vi "ImageCode.vi"() -> ()   [LabVIEW 2012]
uses:
  <vilib>/Rock Robotics/WPI/Camera/WPI_CameraImageSize.ctl
panel:
  out "Image Error Message":string="Timeout in Camera Communications"
  in  "Viewer":enum32{"Camera Image"}(tab)
  in  "Video Enable":bool=TRUE
  out "Output String":string="!195,#END"
  out "Length":i32=9
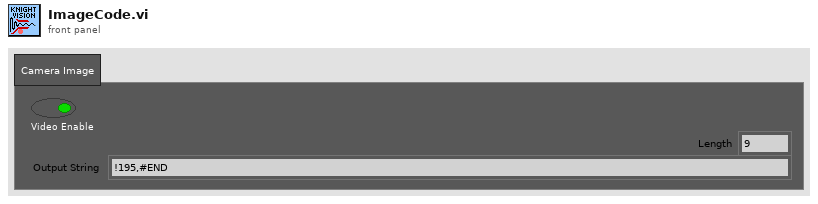
[diagram p1: front panel]
types:
  T1 = typedef "Image Type" = u32
  T2 = typedef "IMAQ Image.ctl" = refnum<image>
  T3 = cluster{"Left":i32, "Top":i32, "Right":i32, "Bottom":i32}
  T4 = typedef "WPI_CameraImageSize.ctl" = enum16{"640x480", "320x240", "160x120"}
  T5 = cluster{"fps":i32, "compression":i32, "Image Size":T4}
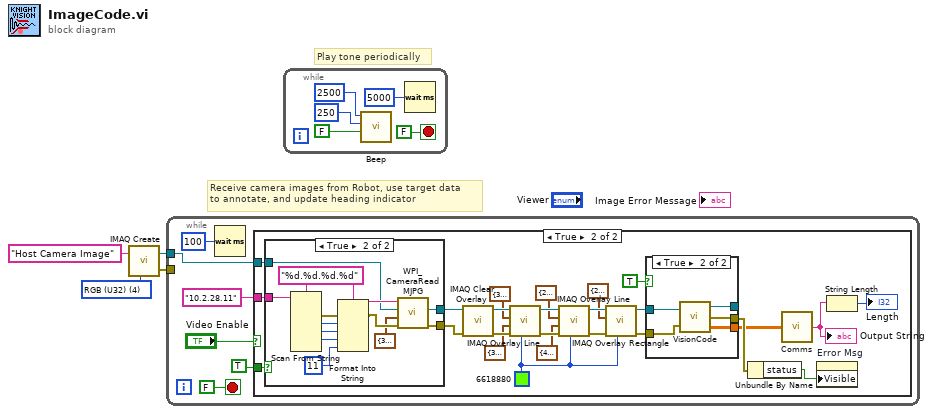
[diagram p0: block diagram]
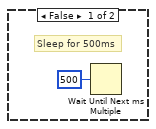
[diagram p2: hidden frame]
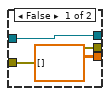
[diagram p3: hidden frame]
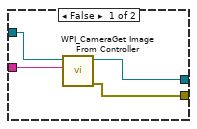
[diagram p4: hidden frame]
diagram:
  w4 = T1 4 items=["Grayscale (U8)", "Grayscale (I16)", "Grayscale (SGL)", "Complex (CSG)", "RGB (U32)", "HSL (U32)", "RGB (U64)"] ("Image Type")
  # "Play tone periodically"
  # "Receive camera images from Robot, use target data\nto annotate, and update heading indicator"
  n1 = call "IMAQ Create"("Image Name"="Host Camera Image", "Image Type"=w4) -> ("New Image"=w2:T2, "error out"=w1:errorcluster)  [unwired: 2 in, 1 out]
  n2 = while {
    tunnel: w2 -> [w8]
    tunnel: w1 -> [_]
    stop <- FALSE stop-if-true
    n3 = Wait (ms)(milliseconds to wait=u32 100) -> ()  [unwired: 1 out]
    n4 = case shown="True" "Video Enable" {
      tunnel: "10.2.28.11" ("Robot IP Address") -> [_ w36]
      tunnel: w8 -> [_ w35]
      tunnel: TRUE -> [_ w32]
      frame False {
        # "Sleep for 500ms"
        n5 = Wait Until Next ms Multiple(millisecond multiple=u32 500) -> ()  [unwired: 1 out]
      }
      frame True {
        w16 = u32 6618880 ("Color")
        n6 = case shown="True" w32 {
          tunnel: w35 -> [w47 w55]
          tunnel: [w45 w53] -> w12
          tunnel: [w46 w54] -> w33
          tunnel: w36 -> [w48 w58]
          frame False {
            n7 = call <vilib>:"WPI_CameraGet Image From Controller.vi"("Controller Address"=w48, "Image"=w47) -> ("error out"=w45:errorcluster, "Image Out"=w46:T2)  [unwired: 2 in, 6 out]
          }
          frame True {
            w50 = "%d.%d.%d.%d" ("format string")
            n8 = Scan From String(format string=w50, input string=w58) -> (error out=w57:errorcluster, output 1=w59:i32, output 2=w60:i32, output 3=w61:i32)  [unwired: 2 in, 7 out]
            n9 = Format Into String(format string=w50, error in=w57, w59, w60, w61, 11 ("IP Suffix:")) -> (resulting string=w56:string, error out=w52:errorcluster)  [unwired: 1 in]
            n10 = call <vilib>:"WPI_CameraRead MJPG.vi"("error in"=w52, "Camera Settings"=T5 {"fps"=30, "compression"=30, "Image Size"=enum."640x480"}, "Image"=w55, "address"=w56) -> ("error out"=w53:errorcluster, "Image Out"=w54:T2)  [unwired: 5 in, 1 out]
          }
        }
        n11 = call "IMAQ Clear Overlay"("error in (no error)"=w12, "Image"=w33) -> ("error out"=w30:errorcluster, "Image Out"=w31:T2)  [unwired: 1 in, 7 out]
        n12 = call "IMAQ Overlay Line"("Color"=w16, "error in (no error)"=w30, "End Point"=cluster{"X":i32, "Y":i32} {"X"=320, "Y"=480}, "Start Point"=cluster{"X":i32, "Y":i32} {"X"=320, "Y"=0}, "Image"=w31) -> ("error out"=w26:errorcluster, "Image Out"=w27:T2)  [unwired: 5 in]
        n13 = call "IMAQ Overlay Line"("Color"=w16, "error in (no error)"=w26, "End Point"=cluster{"X":i32, "Y":i32} {"X"=420, "Y"=240}, "Start Point"=cluster{"X":i32, "Y":i32} {"X"=220, "Y"=240}, "Image"=w27) -> ("error out"=w22:errorcluster, "Image Out"=w23:T2)  [unwired: 5 in]
        n14 = call "IMAQ Overlay Rectangle"("Color"=w16, "error in (no error)"=w22, "Rectangle"=T3 {"Left"=270, "Top"=190, "Right"=370, "Bottom"=290}, "Image"=w23) -> ("error out"=w20:errorcluster, "Image Out"=w18:T2)  [unwired: 6 in]
        n15 = case shown="True" TRUE {
          tunnel: w20 -> [w38 w44]
          tunnel: [w38 w41] -> w19
          tunnel: w18 -> [w39 w43]
          tunnel: [w39 w42] -> _
          tunnel: [dbl[][] [] ("Particle Measurements (Pixels)") w40] -> w15
          frame False {
          }
          frame True {
            n16 = call "VisionCode.vi"("Image Src"=w43, "error in (no error)"=w44) -> ("Image Out"=w42:T2, "error out"=w41:errorcluster, "Particle Measurements (Pixels)"=w40:dbl[][])
          }
        }
        n17 = Unbundle By Name(w19) -> ("status"=w34:bool)
        n18 = call "Comms.vi"("Array"=w15) -> ("String"=w14:string)
        "Output String" <- w14
        n19 = property on="Error Msg" class="Str"("Visible"=w34) -> ()  [unwired: 2 in, 2 out]
        n20 = String Length(string=w14) -> (length=→"Length":i32)
      }
    }
  }
  n21 = while {
    stop <- FALSE stop-if-true
    n22 = call <vilib>:"Beep.vi"("use system alert? (T)"=FALSE, "duration (msec)"=u32 250, "frequency (Hz)"=u32 2500) -> ()  [unwired: 9 in]
    n23 = Wait (ms)(milliseconds to wait=u32 5000) -> ()  [unwired: 1 out]
  }
